vi "Scanner String.vi"(2 "Scanner String (in)":string, 3 "Scanner Settings in":T1={"Scan1"=1, "Scan2"=1, "Scan3"=1, "Scan4"=1, "Scan5"=1, "Scan6"=1, "Scan7"=1, "Scan8"=1, "Scan9"=1, "Scan10"=1, "Scan11"=1, "Scan12"=1, "Scan13"=1, "Scan14"=1, "Scan15"=1, "Scan16"=1} {"Scan16" scale=0.0..2.0; "Scan15" scale=0.0..2.0; "Scan14" scale=0.0..2.0; "Scan13" scale=0.0..2.0; "Scan12" scale=0.0..2.0; "Scan11" scale=0.0..2.0; "Scan10" scale=0.0..2.0; "Scan9" scale=0.0..2.0; "Scan8" scale=0.0..2.0; "Scan7" scale=0.0..2.0; "Scan6" scale=0.0..2.0; "Scan5" scale=0.0..2.0; "Scan4" scale=0.0..2.0; "Scan3" min=0 max=2 scale=0.0..2.0; "Scan2" min=0 max=2 scale=0.0..2.0; "Scan1" min=0 max=2 scale=0.0..2.0}) -> (0 "Scanner Settings out":T1={"Scan1"=1, "Scan2"=1, "Scan3"=1, "Scan4"=1, "Scan5"=1, "Scan6"=1, "Scan7"=1, "Scan8"=1, "Scan9"=1, "Scan10"=1, "Scan11"=1, "Scan12"=1, "Scan13"=1, "Scan14"=1, "Scan15"=1, "Scan16"=1} {"Scan16" scale=0.0..2.0; "Scan15" scale=0.0..2.0; "Scan14" scale=0.0..2.0; "Scan13" scale=0.0..2.0; "Scan12" scale=0.0..2.0; "Scan11" scale=0.0..2.0; "Scan10" scale=0.0..2.0; "Scan9" scale=0.0..2.0; "Scan8" scale=0.0..2.0; "Scan7" scale=0.0..2.0; "Scan6" scale=0.0..2.0; "Scan5" scale=0.0..2.0; "Scan4" scale=0.0..2.0; "Scan3" min=0 max=2 scale=0.0..2.0; "Scan2" min=0 max=2 scale=0.0..2.0; "Scan1" min=0 max=2 scale=0.0..2.0}, 1 "Scanner String (out)":string)   [LabVIEW 2016, in "eec EST 300.lvlib"]
doc: "This utility vi converts the scanner settings cluster into the string used by the instrument."
uses:
  <instrlib>/eec EST 300/eec EST 300.lvlib
  <instrlib>/eec EST 300/Public/Configure/Steps/Low Level/Scanner Settings.ctl
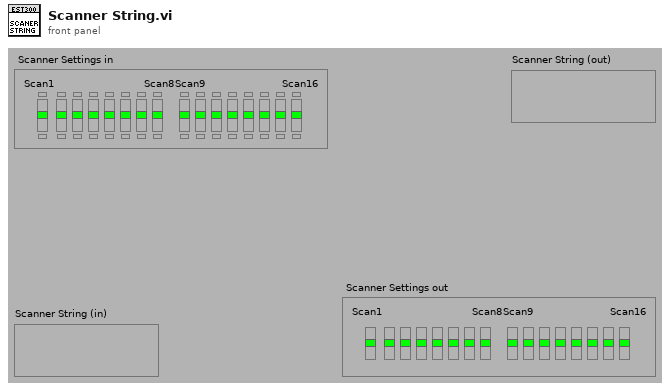
[diagram p1: front panel]
types:
  T1 = typedef "eec EST 300.lvlib/Scanner Settings.ctl" = cluster{"Scan1":i32, "Scan2":i32, "Scan3":i32, "Scan4":i32, "Scan5":i32, "Scan6":i32, "Scan7":i32, "Scan8":i32, "Scan9":i32, "Scan10":i32, "Scan11":i32, "Scan12":i32, "Scan13":i32, "Scan14":i32, "Scan15":i32, "Scan16":i32}
  T2 = cluster{"[0]":i32, "[1]":i32, "[2]":i32, "[3]":i32, "[4]":i32, "[5]":i32, "[6]":i32, "[7]":i32, "[8]":i32, "[9]":i32, "[10]":i32, "[11]":i32, "[12]":i32, "[13]":i32, "[14]":i32, "[15]":i32}
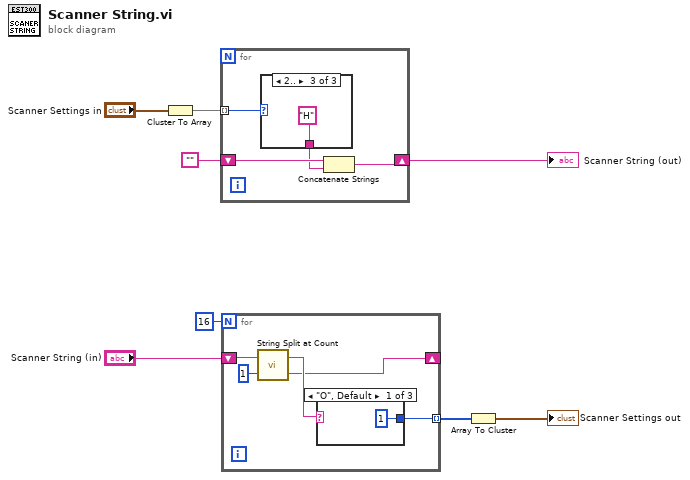
[diagram p0: block diagram]
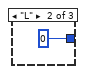
[diagram p2: hidden frame]
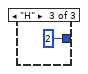
[diagram p3: hidden frame]
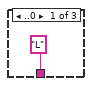
[diagram p4: hidden frame]
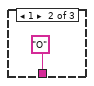
[diagram p5: hidden frame]
diagram:
  n1 = Cluster To Array(cluster="Scanner Settings in") -> (array=w5:i32[])
  n2 = for {
    tunnel: w5 -> [w12] mode=indexing
    shift-right: [w9] -> w7
    shift-left: "" -> [w11]
    n3 = case shown="2.." w12 {
      tunnel: ["L" "O" "H"] -> w10
      frame ..0 {
      }
      frame 1 {
      }
      frame 2.. {
      }
    }
    n4 = Concatenate Strings(w11, w10) -> (w9:string)
  }
  "Scanner String (out)" <- w7
  n5 = for {
    N: 16 -> [_]
    shift-right: [w17] -> _
    shift-left: "Scanner String (in)" -> [w20]
    tunnel: [w16] -> w2 mode=indexing
    n6 = call <instrlib>:"String Split at Count.vi"("# of characters in 1st string"=1, "String to Split"=w20) -> ("2nd String"=w17:string, "1st String"=w18:string)
    n7 = case shown="\"O\", Default" w18 {
      tunnel: [1 0 2] -> w16
      frame "O", Default {
      }
      frame "L" {
      }
      frame "H" {
      }
    }
  }
  n8 = Array To Cluster(array=w2) -> (cluster=→"Scanner Settings out":T2)
